vi "Pulse Stretch.vi"(1 "Stretch (sec)":dbl=1.0, 2 "In":bool) -> (0 "Out":bool)   [LabVIEW 2011]
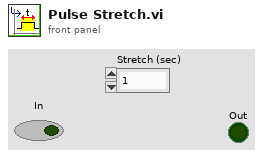
[diagram p1: front panel]
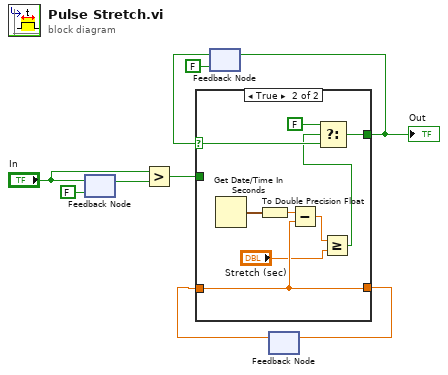
[diagram p0: block diagram]
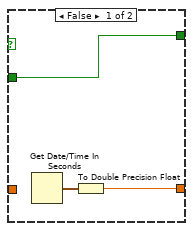
[diagram p2: hidden frame]
diagram:
  n1 = feedback #1(FALSE ("input")) -> (w8:bool)
  n2 = feedback-in #1("In") -> ()
  n3 = Greater?(x="In", y=w8) -> (0:w1:bool)
  n4 = feedback #2(FALSE) -> (w3:bool)
  n5 = feedback #3() -> (w5:dbl)  [unwired: 1 in]
  n6 = case shown="True" w3 {
    selector: w3 -> [_ w16]
    tunnel: [w11 w19] -> w6
    tunnel: w5 -> [_ w19]
    tunnel: [w10 w14] -> w4
    tunnel: w1 -> [w10 _]
    frame False {
      n7 = Get Date/Time In Seconds() -> (seconds since 1Jan1904=w12:timestamp)
      n8 = To Double Precision Float(number=w12) -> (double precision float=w11:dbl)
    }
    frame True {
      n9 = Get Date/Time In Seconds() -> (seconds since 1Jan1904=w21:timestamp)
      n10 = To Double Precision Float(number=w21) -> (double precision float=w20:dbl)
      n11 = Subtract(x=w20, y=w19) -> (x-y=w18:dbl)
      n12 = Greater Or Equal?(x=w18, y="Stretch (sec)") -> (x >= y?=w15:bool)
      n13 = Select(t=FALSE, s=w15, f=w16) -> (s? t:f=w14:bool)
    }
  }
  "Out" <- w4
  n14 = feedback-in #2(w4) -> ()
  n15 = feedback-in #3(w6) -> ()
